vi "image2slopes2phase_test.vi"() -> ()   [LabVIEW 2018]
uses:
  <userlib>/WaveKit.lib/Controls/StatisticsData.ctl
  <userlib>/WaveKit.lib/Controls/HasoSlopes.lvclass
  <userlib>/WaveKit.lib/Classes/Phase/Phase.lvclass
  <userlib>/WaveKit.lib/Classes/Image/Image.lvclass
  <userlib>/WaveKit.lib/Controls/Pupil.lvclass
panel:
  out "Phase values":sgl[][](graph)
  out "Phase statistics":T1
  in  "Camera image file":path=path "D:/SystemAlignment/system_aberation_residual_spots_20191015.himg"
  in  "Haso configuration file":path=path "C:/Program Files (x86)/Imagine Optic/Configuration Files/HASO3_first_7364.dat"
  in  "Filter":u8[](array[numeric])
  out "error out":errorcluster
  in  "error in (no error)":errorcluster
  in  "Output folder":path=path "D:/Data/20200122_Test"
  in  "Output file name":string="test.has"
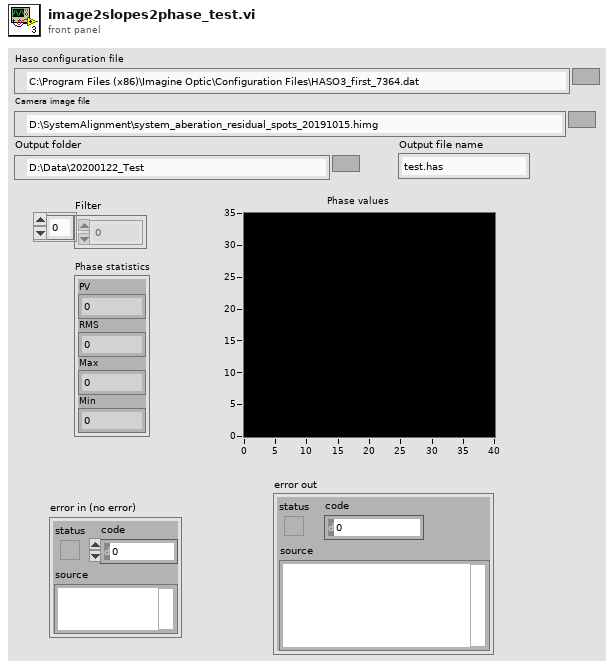
[diagram p1: front panel]
types:
  T1 = typedef "StatisticsData.ctl" = cluster{"PV":sgl, "RMS":dbl, "Max":sgl, "Min":sgl}
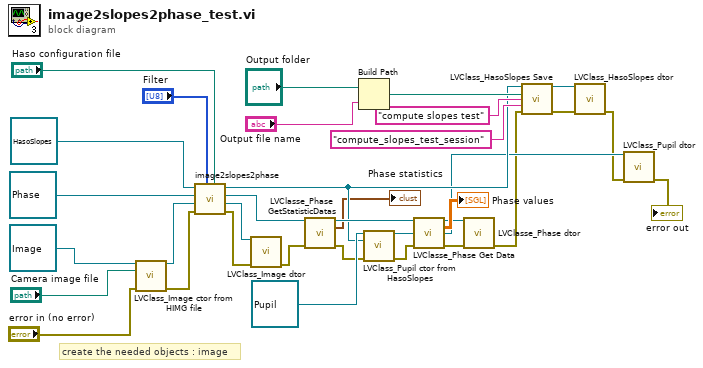
[diagram p0: block diagram]
diagram:
  # "create the needed objects : image"
  n1 = call <userlib>:"LVClass_Image ctor from HIMG file.vi"("Image in"=refnum<class "Image.lvclass"> refnum, "Path to image file"="Camera image file", "error in (no error)"="error in (no error)") -> ("Image out"=w23:refnum<class "Image.lvclass">, "error out"=w22:errorcluster)  [unwired: 11 in]
  n2 = call "image2slopes2phase.vi"("Haso configuration file"="Haso configuration file", "Filter"="Filter", "error in (no error)"=w22, "Image in"=w23, "Phase in"=refnum<class "Phase.lvclass"> refnum, "HasoSlopes in"=refnum<class "HasoSlopes.lvclass"> refnum) -> ("error out"=w18:errorcluster, "Image out"=w17:refnum<class "Image.lvclass">, "Phase out"=w15:refnum<class "Phase.lvclass">, "HasoSlopes out"=w11:refnum<class "HasoSlopes.lvclass">)  [unwired: 2 in]
  n3 = call <userlib>:"LVClass_Image dtor.vi"("Image in"=w17, "error in (no error)"=w18) -> ("error out"=w14:errorcluster)  [unwired: 12 in, 1 out]
  n4 = call <userlib>:"LVClasse_Phase GetStatisticDatas.vi"("Phase in"=w15, "error in (no error)"=w14) -> ("Phase out"=w16:refnum<class "Phase.lvclass">, "StatisticsData"=→"Phase statistics":T1, "error out"=w12:errorcluster)  [unwired: 11 in]
  n5 = Build Path(base path="Output folder", name or relative path="Output file name") -> (appended path=w32:path)
  n6 = call <userlib>:"LVClass_Pupil ctor from HasoSlopes.vi"("Pupil in"=refnum<class "Pupil.lvclass"> refnum, "HasoSlopes.lvclass"=w11, "error in (no error)"=w12) -> ("Pupil out"=w10:refnum<class "Pupil.lvclass">, "error out"=w9:errorcluster)  [unwired: 11 in]
  n7 = call <userlib>:"LVClasse_Phase Get Data.vi"("Phase in"=w16, "Pupil"=w10, "error in (no error)"=w9) -> ("Phase out"=w6:refnum<class "Phase.lvclass">, "data"=→"Phase values":sgl[][], "Pupil (dup)"=w4:refnum<class "Pupil.lvclass">, "error out"=w5:errorcluster)  [unwired: 9 in]
  n8 = call <userlib>:"LVClasse_Phase dtor.vi"("Phase in"=w6, "error in (no error)"=w5) -> ("error out"=w3:errorcluster)  [unwired: 12 in, 1 out]
  n9 = call <userlib>:"LVClass_HasoSlopes Save.vi"("HasoSlopes in"=w11, "path"=w32, "comments"="compute slopes test", "session"="compute_slopes_test_session", "error in (no error)"=w3) -> ("HasoSlopes out"=w19:refnum<class "HasoSlopes.lvclass">, "error out"=w20:errorcluster)  [unwired: 9 in]
  n10 = call <userlib>:"LVClass_HasoSlopes dtor.vi"("HasoSlopes in"=w19, "error in (no error)"=w20) -> ("error out"=w2:errorcluster)  [unwired: 12 in, 1 out]
  n11 = call <userlib>:"LVClass_Pupil dtor.vi"("Pupil in"=w4, "error in (no error)"=w2) -> ("error out"=→"error out":errorcluster)  [unwired: 12 in, 1 out]
